vi "Dynamically Load Reporter.vi"(8 "error in":errorcluster, 10 "Reporter without ext":string) -> (0 "error out":errorcluster, 3 "Approval Tests:Reporter":refnum<class "Reporter.lvclass">)   [LabVIEW 2020, in "Approval Tests.lvlib" / "Reporter.lvclass"]
uses:
  Reporter.lvclass
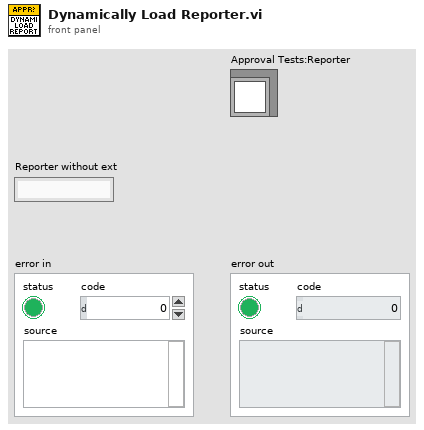
[diagram p1: front panel]
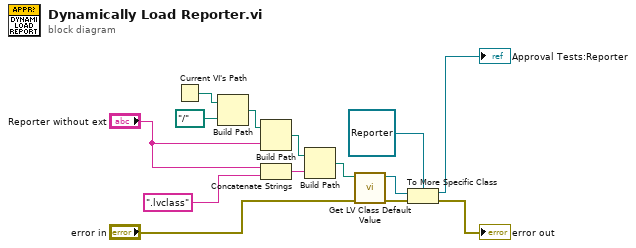
[diagram p0: block diagram]
diagram:
  n1 = Current VI's Path() -> (path=w8:path)
  n2 = Build Path(base path=w8, name or relative path=path "../..") -> (appended path=w6:path)
  n3 = Build Path(base path=w6, name or relative path="Reporter without ext") -> (appended path=w4:path)
  n4 = Concatenate Strings("Reporter without ext", ".lvclass" ("string")) -> (w3:string)
  n5 = Build Path(base path=w4, name or relative path=w3) -> (appended path=w2:path)
  n6 = call <vilib>:"Get LV Class Default Value.vi"("error in (no error)"="error in", "class path"=w2) -> ("error out"=w13:errorcluster, "object"=w1:refnum<class>)  [unwired: 8 in]
  n7 = To More Specific Class(target class=refnum<class "Reporter.lvclass"> refnum ("Approval Tests:Reporter"), reference=w1, error in=w13) -> (specific class reference=→"Approval Tests:Reporter":refnum<class "Reporter.lvclass">, error out=→"error out":errorcluster)
